vi "SVFA Real and Imaginary to Magnitude and Phase (N Ch).vi"(0 "real spectra":cluster{"x0":dbl, "dx":dbl, "real part":dbl[]}[](array[cluster]), 2 "imaginary spectra":T8(array[cluster]), 4 "spectrum info in":T2[](array[typedef]) {"x-axis units" items=["Time (s)"=0, "Frequency-CB (Hz)"=1, "Frequency-CPB (Hz)"=1248, "Frequency-Arbitrary (Hz)"=2357, "Quefrency (s)"=2, "Revolutions (rev)"=3, "Order"=4, "Speed (RPM)"=11, "Speed (rad/s)"=21, "Index"=65535]; "weighting filter" items=["Linear", "A-weighting", "B-weighting", "C-weighting", "ITU-R 468-4", "Dolby", "CCITT", "C-message", "Wb", "Wc", "Wd", "We", "Wf", "Wh", "Wj", "Wk", "Wm", "AES17 20 kHz lowpass", "AES17 40 kHz lowpass", "AES17 20 kHz highpass", "AES17 40 kHz highpass"]; "dB reference [EU]" format="%.2f"; "engineering units" items=["custom..."=0, "V"=1, "A"=21, "C"=30, "pC"=31, "s"=32, "-"=29, "Pa"=2, "N"=20, "g"=3, "m/s^2"=4, "m/s"=5, "m"=6, "mm/s"=12, "mm"=13, "micron/s"=14, "micron"=15, "in/s^2"=7, "in/s"=8, "in"=9, "mil/s"=10, "mil"=11, "rad/s^2"=16, "rad/s"=17, "rad"=18, "deg/s^2"=26, "deg/s"=27, "deg"=28, "RPM"=22, "cycle/s^2"=23, "Hz"=24, "cycle"=25, "strain"=19]; "spectral info"."window" items=["None "=0, "Hanning"=1, "Hamming"=2, "Blackman-Harris"=3, "Exact Blackman"=4, "Blackman"=5, "Flat Top"=6, "4 Term B-Harris "=7, "7 Term B-Harris"=8, "Low Sidelobe"=9, "Force - Exponential"=10, "Gaussian"=62]}, 5 "error in (no error)":errorcluster, 6 "view":T1={"dB On (F)"=FALSE, "unwrap phase (F)"=FALSE, "convert to degree (T)"=TRUE}) -> (14 "magnitude spectra":cluster{"x0":dbl, "dx":dbl, "magnitude":dbl[]}[](array[cluster]), 15 "magnitude unit labels":string[](array[string]), 16 "phase spectra":cluster{"x0":dbl, "dx":dbl, "phase":dbl[]}[](array[cluster]), 17 "phase unit labels":string[](array[string]), 18 "spectrum info out":T2[](array[typedef]) {"x-axis units" items=["Time (s)"=0, "Frequency-CB (Hz)"=1, "Frequency-CPB (Hz)"=1248, "Frequency-Arbitrary (Hz)"=2357, "Quefrency (s)"=2, "Revolutions (rev)"=3, "Order"=4, "Speed (RPM)"=11, "Speed (rad/s)"=21, "Index"=65535]; "weighting filter" items=["Linear", "A-weighting", "B-weighting", "C-weighting", "ITU-R 468-4", "Dolby", "CCITT", "C-message", "Wb", "Wc", "Wd", "We", "Wf", "Wh", "Wj", "Wk", "Wm", "AES17 20 kHz lowpass", "AES17 40 kHz lowpass", "AES17 20 kHz highpass", "AES17 40 kHz highpass"]; "dB reference [EU]" format="%.2f"; "engineering units" items=["custom..."=0, "V"=1, "A"=21, "C"=30, "pC"=31, "s"=32, "-"=29, "Pa"=2, "N"=20, "g"=3, "m/s^2"=4, "m/s"=5, "m"=6, "mm/s"=12, "mm"=13, "micron/s"=14, "micron"=15, "in/s^2"=7, "in/s"=8, "in"=9, "mil/s"=10, "mil"=11, "rad/s^2"=16, "rad/s"=17, "rad"=18, "deg/s^2"=26, "deg/s"=27, "deg"=28, "RPM"=22, "cycle/s^2"=23, "Hz"=24, "cycle"=25, "strain"=19]; "spectral info"."window" items=["None "=0, "Hanning"=1, "Hamming"=2, "Blackman-Harris"=3, "Exact Blackman"=4, "Blackman"=5, "Flat Top"=6, "4 Term B-Harris "=7, "7 Term B-Harris"=8, "Low Sidelobe"=9, "Force - Exponential"=10, "Gaussian"=62]}, 19 "error out":errorcluster)   [LabVIEW 2017]
doc: "Converts spectra from rectangular components to polar components. You can display magnitude and phase information on graphs and send this information to other Spectrum Extended Measurements VIs. Wire data to the <B>real spectrum</B> and <B>imaginary spectrum</B> inputs to determine the polymorphic instance to use or manually select the instance."
uses:
  <vilib>/addons/_NISVFA/_Shared subVIs/Controls/svc_Spectrum Info.ctl
  <vilib>/addons/_NISVFA/_Shared subVIs/Controls/svc_X-Axis Units.ctl
  <vilib>/addons/_NISVFA/_Shared subVIs/Controls/svc_Spectrum Type.ctl
  <vilib>/addons/_NISVFA/_Shared subVIs/Controls/svc_Engineering Units Text Ring.ctl
  <vilib>/addons/_NISVFA/_Shared subVIs/Controls/svc_Weighting Filter Text Ring.ctl
  <vilib>/addons/_NISVFA/_Shared subVIs/Controls/svc_Complimentary Spectrum Units.ctl
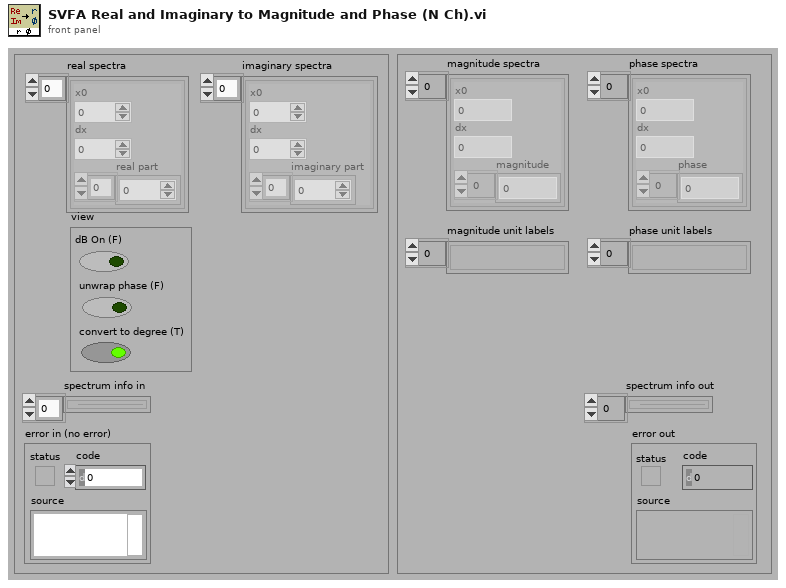
[diagram p1: front panel]
types:
  T1 = cluster{"dB On (F)":bool, "unwrap phase (F)":bool, "convert to degree (T)":bool}
  T2 = typedef "svc_Spectrum Info.ctl" = cluster{"channel name":string, "description":string, "x-axis units":T3, "spectral info":cluster{"spectrum type":T4, "linear/dB":enum16{"linear", "dB"}, "window":u16, "window size":i32, "FFT size":i32}, "engineering units":T5, "custom label":string, "dB reference [EU]":dbl, "peak units":enum16{"rms", "peak", "peak-peak"}, "weighting filter":T6, "spectral density?":bool, "unit label":string, "spectrum skewed?":bool, "complimentary spectrum units":T7}
  T3 = typedef "svc_X-Axis Units.ctl" = u16
  T4 = typedef "svc_Spectrum Type.ctl" = enum16{"FFT Spectrum [complex]", "Amplitude [Magnitude]", "Power [Magnitude^2]", "Cross Spectrum [complex]", "Frequency Response [Complex]"}
  T5 = typedef "svc_Engineering Units Text Ring.ctl" = u16
  T6 = typedef "svc_Weighting Filter Text Ring.ctl" = u16
  T7 = typedef "svc_Complimentary Spectrum Units.ctl" = enum16{"none", "radians", "degrees", "cycles", "imaginary"}
  T8 = cluster{"x0":dbl, "dx":dbl, "imaginary part":dbl[]}[]
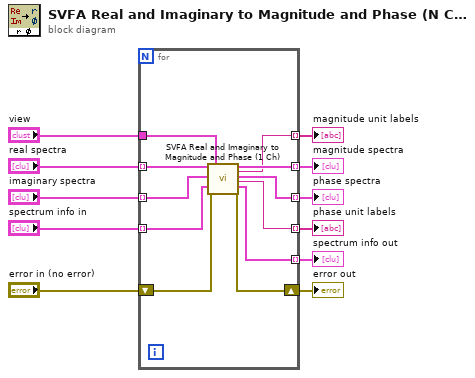
[diagram p0: block diagram]
diagram:
  n1 = for {
    tunnel: [w13] -> w2 mode=indexing
    tunnel: "real spectra" -> [w16] mode=indexing
    tunnel: "imaginary spectra" -> [w17] mode=indexing
    tunnel: [w15] -> w9 mode=indexing
    tunnel: [w14] -> w7 mode=indexing
    tunnel: [w18] -> w6 mode=indexing
    tunnel: "spectrum info in" -> [w22] mode=indexing
    tunnel: [w19] -> w4 mode=indexing
    shift-right: [w20] -> w8
    shift-left: "error in (no error)" -> [w21]
    tunnel: "view" -> [w12]
    n2 = call <vilib>:"SVFA Real and Imaginary to Magnitude and Phase (1 Ch).vi"("real spectrum"=w16, "imaginary spectrum"=w17, "spectrum info in"=w22, "error in (no error)"=w21, "view"=w12) -> ("magnitude spectrum"=w15:cluster{"x0":dbl, "dx":dbl, "magnitude":dbl[]}, "magnitude unit label"=w13:string, "phase spectrum"=w14:cluster{"x0":dbl, "dx":dbl, "phase":dbl[]}, "phase unit label"=w19:string, "spectrum info out"=w18:T2, "error out"=w20:errorcluster)  [unwired: 9 in]
  }
  "magnitude spectra" <- w9
  "phase spectra" <- w7
  "error out" <- w8
  "spectrum info out" <- w6
  "phase unit labels" <- w4
  "magnitude unit labels" <- w2
